vi "StartTrial.vi"(8 "error in (no error)":errorcluster, 11 "TrialBasedExperiment in":refnum<class "PassiveFixation.lvclass">) -> (0 "error out":errorcluster, 3 "TrialBasedExperiment out":refnum<class "PassiveFixation.lvclass">)   [LabVIEW 2010, in "PassiveFixation.lvclass"]
uses:
  PassiveFixation.lvclass
  PassiveExperiment/PassiveExperiment.lvclass
  Matlab API/Matlab API.lvlib
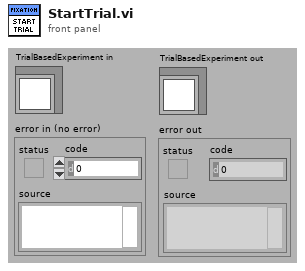
[diagram p1: front panel]
types:
  T1 = cluster{"Intertrial":dbl, "AcquireFixation":dbl, "HoldFixation":dbl, "DelayPeriod":dbl, "ResponsePeriod":dbl}
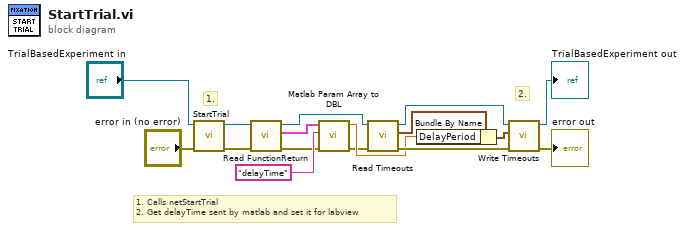
[diagram p0: block diagram]
diagram:
  # "2."
  # "1. Calls netStartTrial\n2. Get delayTime sent by matlab and set it for labview"
  # "1."
  n1 = call-parent "StartTrial.vi"("error in (no error)"="error in (no error)", "TrialBasedExperiment in"="TrialBasedExperiment in") -> ("error out"=w11:errorcluster, "TrialBasedExperiment out"=w14:refnum<class "PassiveFixation.lvclass">)  [unwired: 8 in]
  n2 = call-dynamic "Read FunctionReturn.vi"("error in (no error)"=w11, "MatlabExperiment in"=w14) -> ("error out"=w4:errorcluster, "FunctionReturn"=w9:cluster{"Name":string, "Data":variant}[], "MatlabExperiment out"=w13:refnum<class "PassiveFixation.lvclass">)  [unwired: 7 in]
  n3 = call "Matlab Param Array to DBL.vi"("error in (no error)"=w4, "Name"="delayTime", "Matlab Param Array"=w9) -> ("error out"=w3:errorcluster, "data"=w6:dbl)  [unwired: 7 in]
  n4 = call-dynamic "Read Timeouts.vi"("error in (no error)"=w3, "TrialBasedExperiment in"=w13) -> ("error out"=w10:errorcluster, "Timeouts"=w7:T1, "TrialBasedExperiment out"=w12:refnum<class "PassiveFixation.lvclass">)  [unwired: 7 in]
  n5 = Bundle By Name(cluster=w7, "DelayPeriod"=w6) -> (w5:T1)
  n6 = call-dynamic "Write Timeouts.vi"("error in (no error)"=w10, "Timeouts"=w5, "TrialBasedExperiment in"=w12) -> ("error out"=→"error out":errorcluster, "TrialBasedExperiment out"=→"TrialBasedExperiment out":refnum<class "PassiveFixation.lvclass">)  [unwired: 7 in]
